vi "VariantToStr.vi"(1 "COM":refnum<visa-resource-name>) -> (0 "ComStr":string)   [LabVIEW 2013]
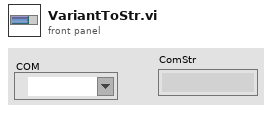
[diagram p1: front panel]
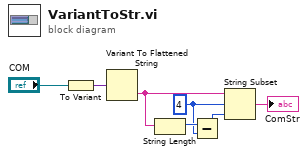
[diagram p0: block diagram]
diagram:
  w4 = 4 ("偏移量(0)")
  n1 = To Variant(anything="COM") -> (Variant=w7:variant)
  n2 = Variant To Flattened String(Variant=w7) -> (data string=w6:string)  [unwired: 1 out]
  n3 = String Length(string=w6) -> (length=w5:i32)
  n4 = Subtract(x=w5, y=w4) -> (x-y=w3:i32)
  n5 = String Subset(string=w6, offset (0)=w4, length (rest)=w3) -> (substring=→"ComStr":string)
